vi "Initialize Workspace Object.vi"(8 "error in (no error)":errorcluster, 11 "State":T1) -> (0 "error out":errorcluster)   [LabVIEW 2023, in "J1939 Workspace Shared.lvlib"]
uses:
  J1939 Workspace Shared.lvlib
  Types/UI.StateVariables.ctl
  <vilib>/NI VeriStand/Display Template Support/DisplayTemplateSupport.llb/enum_Display Template Handler Minimal To Widget Msg.ctl
  <vilib>/NI VeriStand/Execution/Workspace/SystemStateRegEventRef.ctl
  <vilib>/NI VeriStand/Execution/Workspace/Target State Info.ctl
  <vilib>/NI VeriStand/Execution/Workspace/Target State.ctl
  Types/Private Data.ctl
  <vilib>/NI/STM/TCP/TCP Connection Info.ctl
  <vilib>/NI/STM/SubVIs/MetaDataElement.ctl
  Addon/Addon Shared/Types/Error Cluster.ctl
  Addon/Addon Shared/Types/Error Types.ctl
  NationalInstruments.VeriStand.SystemStorage
  <vilib>/NI VeriStand/Display Template Support/DisplayTemplateSupport.llb/enum_Display Template Handler Minimal To Workspace.ctl
  <vilib>/NI VeriStand/Execution/Workspace/WorkspaceAPI.ctl
  NationalInstruments.VeriStand.ClientAPI
  <vilib>/NI VeriStand/Execution/Workspace/SystemStateEventRef.ctl
  Types/UI.Refs.ctl
  SubModules/CAN-Streaming-Support/Source/Addon/Addon Shared/Types/Type Filter.ctl
  SubModules/CAN-Streaming-Support/Source/Addon/Addon Shared/Types/Direction Filter.ctl
  SubModules/CAN-Streaming-Support/Source/UIs/Workspace Shared/Types/Host Stream Queue Refs.ctl
  SubModules/CAN-Streaming-Support/Source/UIs/Workspace Shared/Types/Host Stream Queue Type.ctl
  SubModules/CAN-Streaming-Support/Source/UIs/Workspace Shared/Types/Host Stream Queue Command.ctl
  <vilib>/xnet/xnet.llb/XNET Frame CAN.ctl
  <vilib>/xnet/xnet.llb/XNET Frame Type CAN.ctl
  <vilib>/Utility/miscctls.llb/LVStringsAndValuesArrayTypeDef_U8.ctl
  Addon/Addon Shared/J1939 Addon Shared.lvlib
  <vilib>/NI/STM/NI STM.lvlib
  <vilib>/NI VeriStand/Execution/Workspace/NI_VS Workspace ExecutionAPI.lvlib
  SubModules/CAN-Streaming-Support/Source/Addon/Addon Shared/CAN Stream Support Shared.lvlib
  SubModules/CAN-Streaming-Support/Source/UIs/Workspace Shared/CAN Stream Support Workspace Shared.lvlib
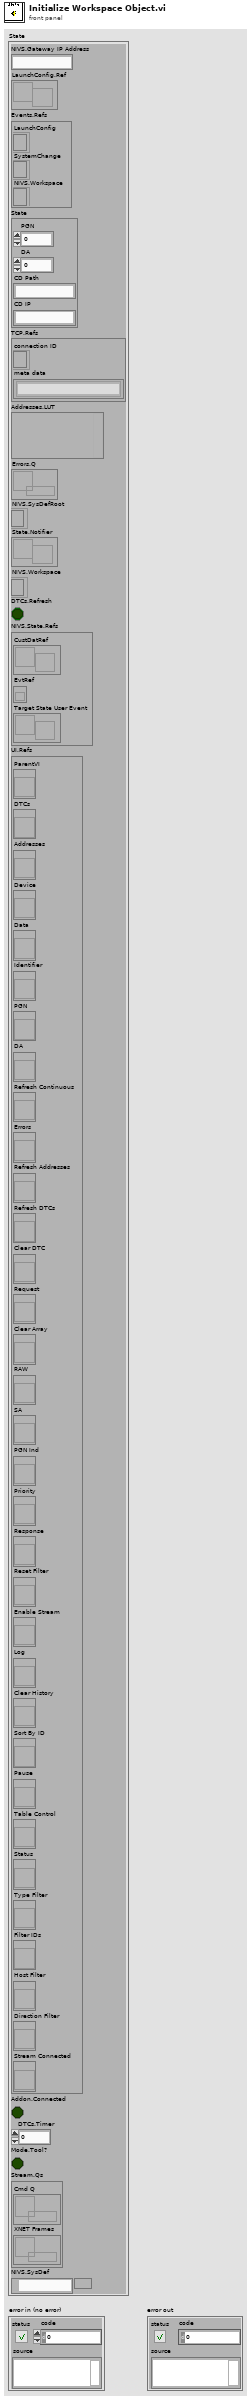
[diagram p1: front panel]
types:
  T1 = typedef "J1939 Workspace Shared.lvlib/UI.StateVariables.ctl" = cluster{"NIVS.Gateway IP Address":string, "LaunchConfig.Ref":refnum<user-event>, "Events.Refs":cluster{"LaunchConfig":refnum<event-registration>, "SystemChange":T2, "NIVS.Workspace":refnum<event-registration>}, "State":T3, "TCP.Refs":T4, "Addresses.LUT":variant, "Errors.Q":refnum<queue>, "NIVS.SysDefRoot":refnum<k24>, "State.Notifier":refnum<user-event>, "NIVS.Workspace":T6, "DTCs.Refresh":bool, "NIVS.State.Refs":T7, "UI.Refs":T8, "Addon.Connected":bool, "DTCs.Timer":u32, "Mode.Tool?":bool, "Stream.Qs":T9, "NIVS.SysDef":path}
  T2 = typedef "NI_VS Workspace ExecutionAPI.lvlib/SystemStateRegEventRef.ctl" = refnum<event-registration>
  T3 = typedef "J1939 Workspace Shared.lvlib/Private Data.ctl" = cluster{"PGN":u32, "DA":u8, "CD Path":string, "CD IP":string}
  T4 = typedef "NI STM.lvlib/TCP Connection Info.ctl" = cluster{"connection ID":refnum<k5>, "meta data":T5[]}
  T5 = typedef "NI STM.lvlib/MetaDataElement.ctl" = string
  T6 = typedef "NI_VS Workspace ExecutionAPI.lvlib/WorkspaceAPI.ctl" = refnum<k24>
  T7 = typedef "NI_VS Workspace ExecutionAPI.lvlib/SystemStateEventRef.ctl" = cluster{"CustDatRef":refnum<user-event>, "EvtRef":refnum<k27>, "Target State User Event":refnum<user-event>}
  T8 = typedef "J1939 Workspace Shared.lvlib/UI.Refs.ctl" = cluster{"ParentVI":refnum<vi>, "DTCs":refnum<vi>, "Addresses":refnum<vi>, "Device":refnum<vi>, "Data":refnum<vi>, "Identifier":refnum<vi>, "PGN":refnum<vi>, "DA":refnum<vi>, "Refresh Continuous":refnum<vi>, "Errors":refnum<vi>, "Refresh Addresses":refnum<vi>, "Refresh DTCs":refnum<vi>, "Clear DTC":refnum<vi>, "Request":refnum<vi>, "Clear Array":refnum<vi>, "RAW":refnum<vi>, "SA":refnum<vi>, "PGN Ind":refnum<vi>, "Priority":refnum<vi>, "Response":refnum<vi>, "Reset Filter":refnum<vi>, "Enable Stream":refnum<vi>, "Log":refnum<vi>, "Clear History":refnum<vi>, "Sort By ID":refnum<vi>, "Pause":refnum<vi>, "Table Control":refnum<vi>, "Status":refnum<vi>, "Type Filter":refnum<vi>, "Filter IDs":refnum<vi>, "Host Filter":refnum<vi>, "Direction Filter":refnum<vi>, "Stream Connected":refnum<vi>}
  T9 = typedef "CAN Stream Support Workspace Shared.lvlib/Host Stream Queue Refs.ctl" = cluster{"Cmd Q":refnum<queue>, "XNET Frames":refnum<queue>}
  T10 = enum8{"Enabled", "Disabled", "Disabled and Grayed Out"}
  T11 = typedef "LVStringsAndValuesArrayTypeDef_U8.ctl" = cluster{"String":string, "Value":u8}[]
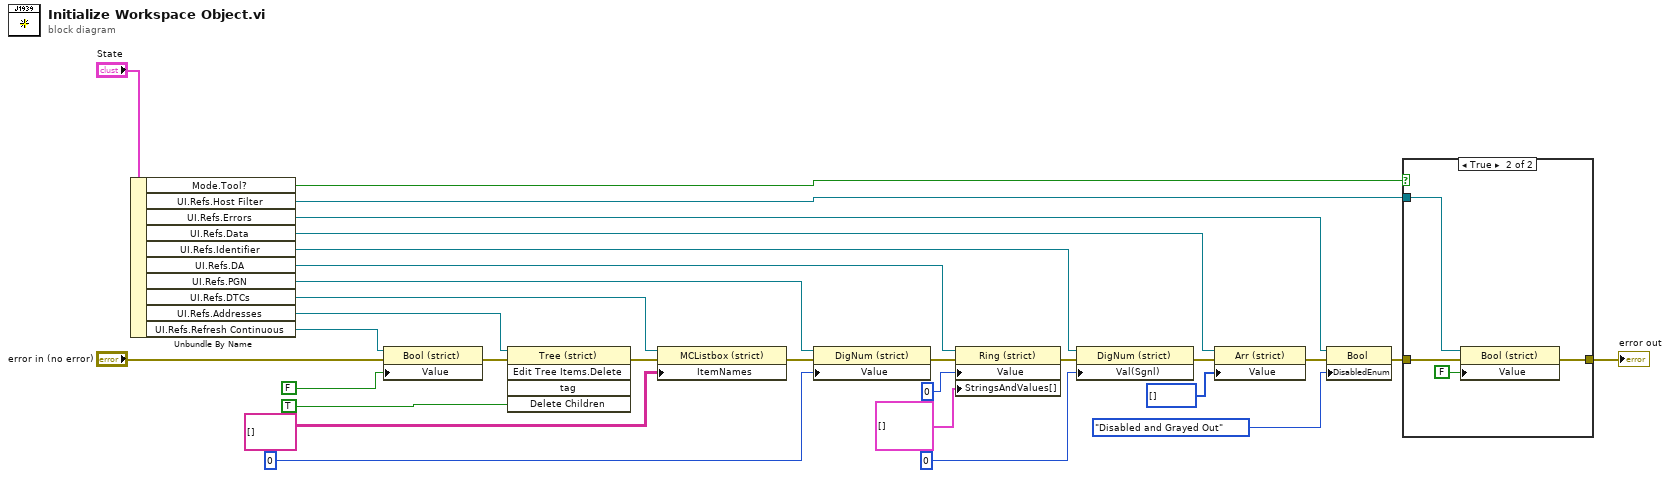
[diagram p0: block diagram]
diagram:
  n1 = Unbundle By Name("State") -> ("Mode.Tool?"=w1:bool, "UI.Refs.Host Filter"=w2:refnum<vi>, "UI.Refs.Errors"=w29:refnum<vi>, "UI.Refs.Data"=w23:refnum<vi>, "UI.Refs.Identifier"=w19:refnum<vi>, "UI.Refs.DA"=w17:refnum<vi>, "UI.Refs.PGN"=w14:refnum<vi>, "UI.Refs.DTCs"=w11:refnum<vi>, "UI.Refs.Addresses"=w8:refnum<vi>, "UI.Refs.Refresh Continuous"=w7:refnum<vi>)
  n2 = property class="Bool (strict)"(reference=w7, error in="error in (no error)", "Value"=FALSE) -> (error out=w10:errorcluster)  [unwired: 1 out]
  n3 = invoke class="Tree (strict)" method="Edit Tree Items.Delete"(reference=w8, error in=w10, "Delete Children"=TRUE ("Delete Children?")) -> (error out=w13:errorcluster)  [unwired: 2 in, 4 out]
  n4 = property class="MCListbox (strict)"(reference=w11, error in=w13, "ItemNames"=string[][] [] ("Item Names")) -> (error out=w16:errorcluster)  [unwired: 1 out]
  n5 = property class="DigNum (strict)"(reference=w14, error in=w16, "Value"=u32 0) -> (error out=w18:errorcluster)  [unwired: 1 out]
  n6 = property class="Ring (strict)"(reference=w17, error in=w18, "Value"=u8 0, "StringsAndValues[]"=T11 [] ("Strings And Values []")) -> (error out=w20:errorcluster)  [unwired: 1 out]
  n7 = property class="DigNum (strict)"(reference=w19, error in=w20, "Val(Sgnl)"=u32 0 ("Value (Signaling)")) -> (error out=w24:errorcluster)  [unwired: 1 out]
  n8 = property class="Arr (strict)"(reference=w23, error in=w24, "Value"=u8[] []) -> (error out=w27:errorcluster)  [unwired: 1 out]
  n9 = property class="Bool"(reference=w29, error in=w27, "DisabledEnum"=T10."Disabled and Grayed Out" ("f")) -> (error out=w4:errorcluster)  [unwired: 1 out]
  n10 = case shown="True" w1 {
    tunnel: w4 -> [w31 w35]
    tunnel: [w31 w34] -> w3
    tunnel: w2 -> [_ w33]
    frame False {
    }
    frame True {
      n11 = property class="Bool (strict)"(reference=w33, error in=w35, "Value"=FALSE) -> (error out=w34:errorcluster)  [unwired: 1 out]
    }
  }
  "error out" <- w3
